vi "Assign 3 Seat belt warning system (2).vi"() -> ()   [LabVIEW 2021]
panel:
  out "warning light":bool
  in  "ignition_on":bool
  in  "buckled up":bool
  in  "driver present":bool
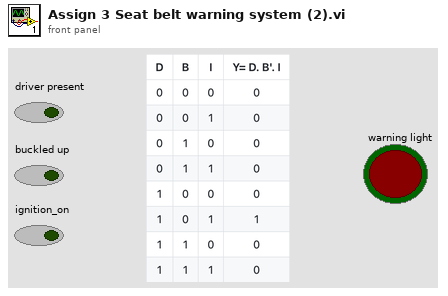
[diagram p1: front panel]
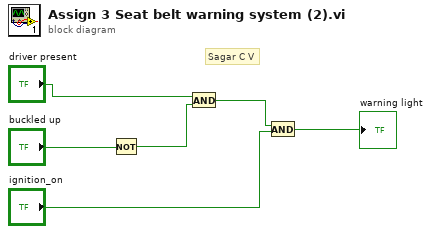
[diagram p0: block diagram]
diagram:
  # "Sagar C V"
  n1 = Not(x="buckled up") -> (.not. x?=w1:bool)
  n2 = And(x="driver present", y=w1) -> (x .and. y?=w6:bool)
  n3 = And(x=w6, y="ignition_on") -> (x .and. y?=→"warning light":bool)
